vi "_PC_Pub pyErrorLineCorrection.vi"(2 "error in (no error)":errorcluster, 3 "scriptStartIdx":i32) -> (0 "error out":errorcluster)   [LabVIEW 2018]
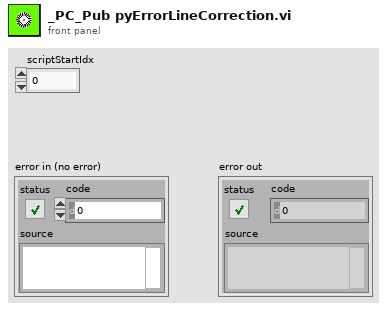
[diagram p1: front panel]
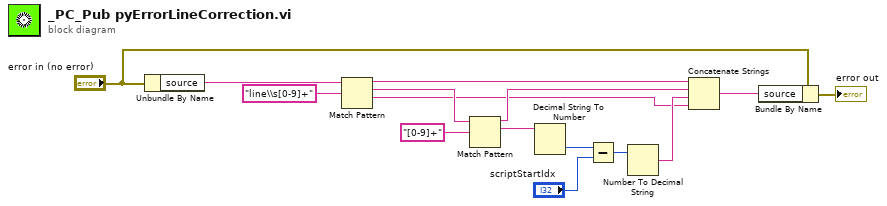
[diagram p0: block diagram]
diagram:
  n1 = Unbundle By Name("error in (no error)") -> ("source"=w15:string)
  n2 = Match Pattern(string=w15, regular expression="line\\s[0-9]+") -> (before substring=w8:string, match substring=w13:string, after substring=w5:string)  [unwired: 1 in, 1 out]
  n3 = Match Pattern(string=w13, regular expression="[0-9]+") -> (before substring=w7:string, match substring=w11:string)  [unwired: 1 in, 2 out]
  n4 = Decimal String To Number(string=w11) -> (number=w4:i32)  [unwired: 2 in, 1 out]
  n5 = Subtract(x=w4, y="scriptStartIdx") -> (x-y=w9:i32)
  n6 = Number To Decimal String(number=w9) -> (decimal integer string=w6:string)  [unwired: 1 in]
  n7 = Concatenate Strings(w8, w7, w6, w5) -> (w3:string)
  n8 = Bundle By Name(cluster="error in (no error)", "source"=w3) -> (→"error out":errorcluster)
